vi "Set Bitmap.vi"(8 "error in (no error)":errorcluster, 10 "Bitmap":u32[][](array[numeric]), 11 "Glyph Canvas in":refnum<class "Glyph Canvas.lvclass">) -> (0 "error out":errorcluster, 3 "Glyph Canvas out":refnum<class "Glyph Canvas.lvclass">)   [LabVIEW 2020, in "Glyph Drawer.lvlib" / "Glyph Canvas.lvclass"]
uses:
  Glyph Canvas.lvclass
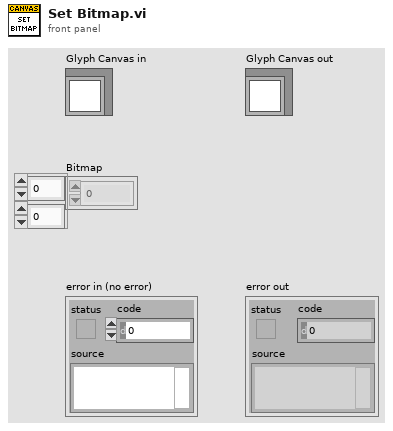
[diagram p1: front panel]
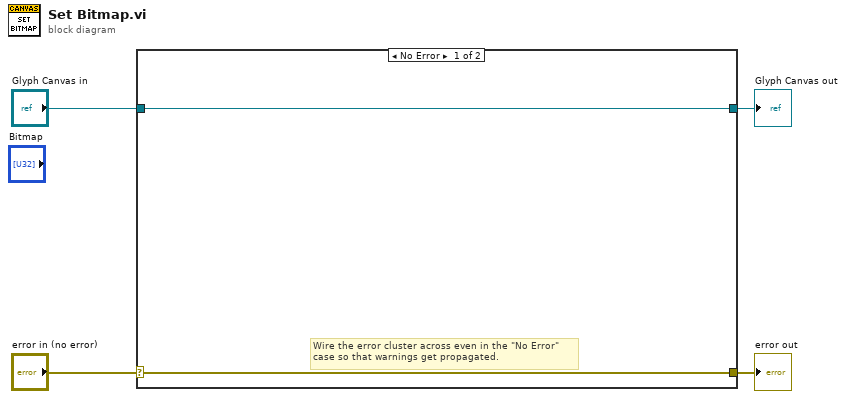
[diagram p0: block diagram]
diagram:
  n1 = case shown="No Error" "error in (no error)" {
    selector: "error in (no error)" -> [w5 w8]
    tunnel: [w5 w8] -> w3
    tunnel: [w6 w7] -> w1
    tunnel: "Glyph Canvas in" -> [w6 w7]
    frame No Error {
      # "Wire the error cluster across even in the \"No Error\"\ncase so that warnings get propagated."
    }
    frame Error {
    }
  }
  "error out" <- w3
  "Glyph Canvas out" <- w1
